vi "Query Arduino Moving Status.vi"(8 "error in (no error)":errorcluster, 10 "motor (0:n-1)":i32, 11 "VISA resource name":refnum<visa-resource-name>) -> (0 "error out":errorcluster, 1 "moving?":bool, 2 "m":i32, 3 "reference out":refnum<visa-resource-name>, 4 "response":string)   [LabVIEW 2022 SP3]
uses:
  <vilib>/regexp/Match Regular Expression.xnode
  FW Arduino Control.lvclass
panel:
  in  "error in":errorcluster
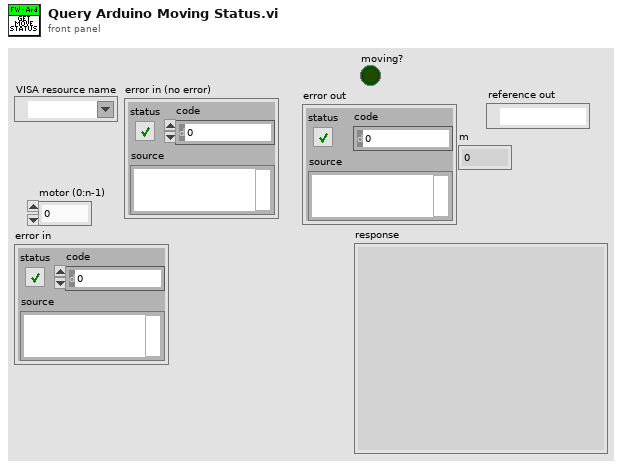
[diagram p1: front panel]
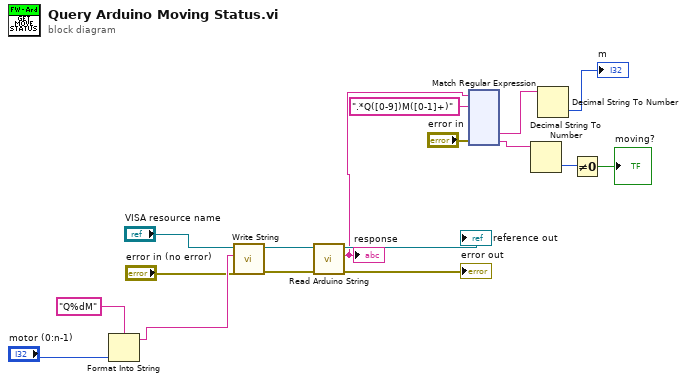
[diagram p0: block diagram]
diagram:
  n1 = Format Into String(format string="Q%dM", "motor (0:n-1)") -> (resulting string=w13:string)  [unwired: 2 in, 1 out]
  n2 = call "Write String.vi"("error in (no error)"="error in (no error)", "String"=w13, "VISA resource name"="VISA resource name") -> ("error out"=w16:errorcluster, "VISA resource name out"=w17:refnum<visa-resource-name>)  [unwired: 7 in]
  n3 = call "Read Arduino String.vi"("error in (no error)"=w16, "reference"=w17) -> ("error out"=→"error out":errorcluster, "response"=w6:string, "reference out"=→"reference out":refnum<visa-resource-name>)  [unwired: 7 in]
  "response" <- w6
  n4 = xnode "Match Regular Expression"("input string"=w6, "regular expression"=".*Q([0-9])M([0-1]+)", "error in"="error in") -> ("submatch 1"=w5:string, "submatch 2"=w3:string)  [unwired: 3 in, 5 out]
  n5 = Decimal String To Number(string=w3) -> (number=w2:i32)  [unwired: 2 in, 1 out]
  n6 = Decimal String To Number(string=w5) -> (number=→"m":i32)  [unwired: 2 in, 1 out]
  n7 = Not Equal To 0?(x=w2) -> (x != 0?=→"moving?":bool)
